vi "BlockPossibleShot.vi"(8 "error in (no error)":errorcluster, 9 "Game ref":refnum<class "Game.lvclass">, 10 "Robot in":refnum<class "Robot.lvclass">, 11 "DefendGoalTactic in":refnum<class "DefendGoalTactic.lvclass">) -> (0 "error out":errorcluster, 2 "Robot out":refnum<class "Robot.lvclass">, 3 "DefendGoalTactic out":refnum<class "DefendGoalTactic.lvclass">)   [LabVIEW 2023, in "DefendGoalTactic.lvclass"]
uses:
  DefendGoalTactic.lvclass
  Game_class/Game.lvclass
  Robot_class/Robot.lvclass
  Game_class/Game.lvclass/Game.ctl
  Object_class/Object.lvclass/Object.ctl
  Field_class/Field.lvclass/Field.ctl
  Robot_class/Robot.lvclass/Robot.ctl
  Game_class/Read BallRef.vi
  Game_class/Read FieldRef.vi
  Field_class/Read ourGoalPosition.vi
  Object_class/Read position(x,y).vi
  Robot_class/Write dest_orientation.vi
  Robot_class/Write dest_x.vi
  Robot_class/Write dest_y.vi
  Ball_class/Ball.lvclass
  C:/Users/ebert/Desktop/roboime/SSL_AI/Object_class/Object.lvclass
  Field_class/Field.lvclass
  <vilib>/Analysis/NI_AALPro.lvlib
  Utilities_class/Utilities.lvclass
  <vilib>/Analysis/coordinate.llb/2D Cartesian Coordinate Rotation (Scalar).vi
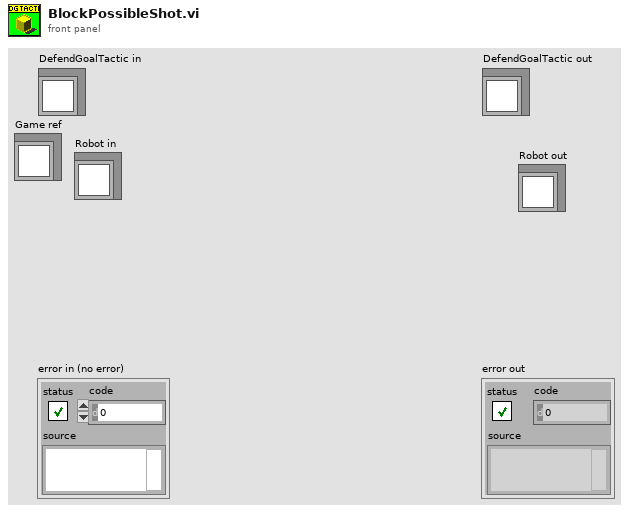
[diagram p1: front panel]
types:
  T1 = typedef "NewParameters.ctl" = cluster{"PenaltyDistance":dbl, "DistanceAttackerToBackBall":dbl, "Division":enum16{"Div B", "Div A"}, "DistanceToAvoidyEnemyRobot":dbl, "BallPlacementDistance":dbl, "DisatanceBehindBallToStealBall":dbl, "MaxDistanceToPositionKickoff":dbl, "BlockEnemyTarget":bool, "MaxStopVAng":dbl, "DistanceMarkerToEnemy":dbl, "IgnoreDribblerContact":bool, "DistanceToBeginEnemyPosession":dbl, "GoToBallWhenEnemyNotMoving":bool, "EnemyDistanceToReduceVelocity":dbl, "TurnOnEnemyDistanceToReduceVelocity":bool, "EnemyDistanceToShootOutBall":dbl, "DefenseKickBall":bool, "MoreKickToGoal? (0-0.3)":dbl, "ChipKickInEnemyField":bool, "ShootOutRobotId":dbl, "FieldLenghtDenominatorInShootOut":dbl, "AdjustPositionInBallPlacement":bool, "PowerGodPass":dbl, "VelocityAbortEnemyPos":dbl, "MaxDistToBeginPass":dbl, "MinDistToBeginPass":dbl, "VelocityInDirects":dbl, "BadDribblerIDs":i32[], "NewKickToDistanceAroundBall":dbl, "PowerAvoidColisionMarker":dbl, "DistanceToAvoidColisionMarker":dbl, "AvoidBallKick":dbl, "DistanceTryKick":dbl, "SuicideKickDIstance":dbl, "AdjustFirstKickDistance":dbl, "AvoidAimLessKick":dbl, "DistanceToAvoidyEnemyShootRobot ":dbl, "NumberOfMarkers":dbl, "PotField":bool, "PIDLateral":bool, "MinDistanceFirstKickX":dbl, "MinDistanceFirstKickY":dbl, "FractionOfDistToTouchGround\nAfterChipKick":dbl, "FractionOfKickxWhen\nComposedWithKickz":dbl, "Style":T2, "MoveInTurnState":bool, "DistFromEnemyToConsider\nMoveInTurnState":dbl, "CascadePID":bool, "TurnAroundParameters":cluster{"Radius":dbl, "Multiplier":dbl, "ChordAngle":dbl}, "SafeDriveVel":dbl, "DistanceToGoToBackBall":dbl, "minDistanceToNotFinish\nEnemyPossession":dbl, "OneTouchShot":cluster{"angleFactor":dbl, "maxAngle":dbl, "Attack":bool, "Defense":bool}, "OpenAngleToGoal":cluster{"minAngle":dbl, "maxAngle":dbl, "minEvaluation":dbl}, "ShotInterception":cluster{"shotSpeed":dbl, "minEnemySpeed":dbl, "maxEnemySpeed":dbl, "minEvaluation":dbl}, "AllyTeamArray":T3[], "maxDefendersNumber":i32, "Zone":cluster{"GuardPositionArray":dbl[][], "ZoneMidField":dbl[], "CenterForwardWidth":dbl}, "MinEvaluationToShoot":dbl, "PassInterception":cluster{"maxPassSpeed":dbl, "minPassSpeed":dbl, "minEnemySpeed":dbl, "chipPassDistance":dbl, "chipPassEvaluation":dbl, "minEvaluation":dbl, "maxEnemySpeed":dbl}, "PassDistance":cluster{"maxDistance":dbl, "minDistance":dbl}, "receiverSpeed":dbl, "maxBallSpeed":dbl, "slackTime":dbl, "Turning radius":dbl, "Turning v_ang":dbl, "AlignError":cluster{"Distance":dbl, "Orientation":dbl, "V_norm(m/s)":dbl, "V_ang (rad/s)":dbl}, "RobotRadius":dbl, "KickerDistance":dbl, "keeper angle  to cover goalpost":dbl}
  T2 = typedef "Style.ctl" = enum16{"Insanity", "Offensive", "Defensive"}
  T3 = typedef "AllyTeam.ctl" = enum16{"Keeper", "Defender", "Attacker"}
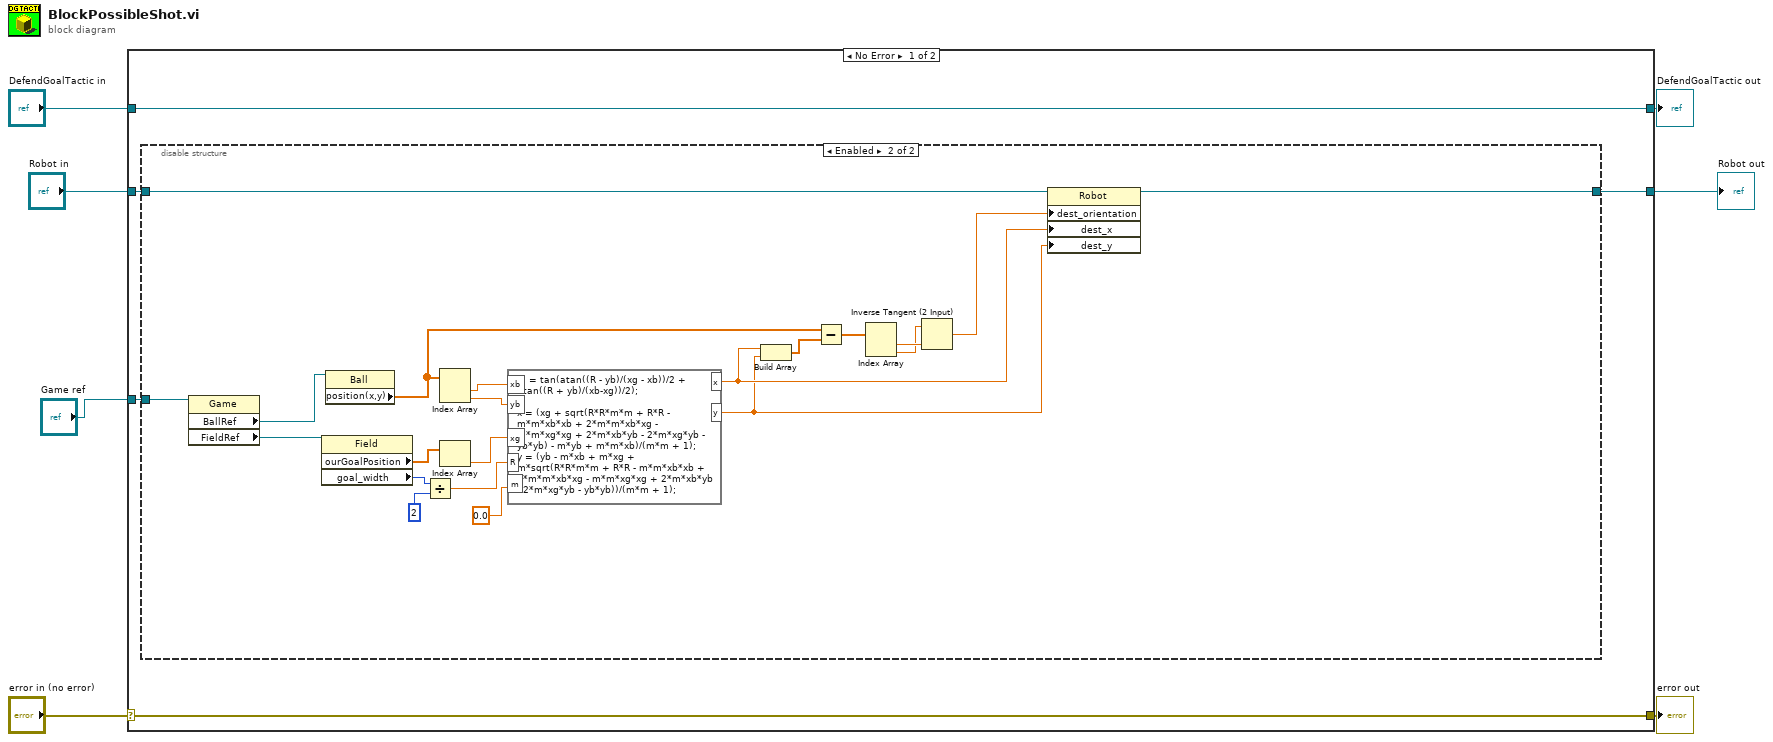
[diagram p0: block diagram]
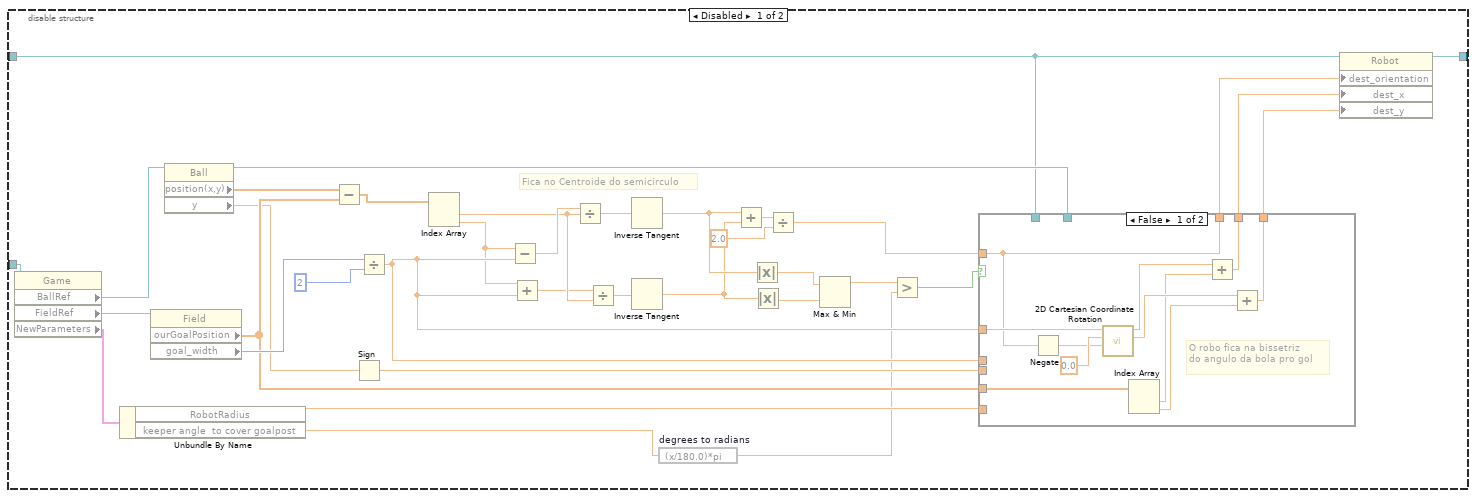
[diagram p2: hidden frame]
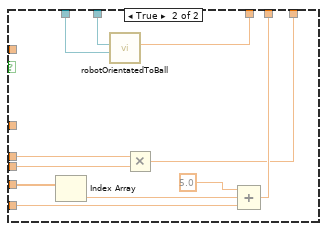
[diagram p3: hidden frame]
diagram:
  n1 = case shown="No Error" "error in (no error)" {
    selector: "error in (no error)" -> [w11 w94]
    tunnel: [w11 w94] -> w6
    tunnel: [w12 w93] -> w4
    tunnel: "DefendGoalTactic in" -> [w12 w93]
    tunnel: "Game ref" -> [w10 _]
    tunnel: "Robot in" -> [w8 w92]
    tunnel: [w9 w92] -> w1
    frame No Error {
      n2 = disable-structure shown="Enabled" {
        disable-tunnel: w10 -> [w23 w91]
        disable-tunnel: [w22 w75] -> w9
        disable-tunnel: w8 -> [w21 w76]
        frame Disabled {
          # "Fica no Centroide do semicirculo"
          n3 = property class="Game"(reference=w23) -> ("BallRef"=w48:refnum<class "Ball.lvclass">, "FieldRef"=w47:refnum<class "Field.lvclass">, "NewParameters"=w29:T1)  [unwired: 1 in, 2 out]
          n4 = Unbundle By Name(w29) -> ("RobotRadius"=w28:dbl, "keeper angle  to cover goalpost"=w13:dbl)
          n5 = property class="Field"(reference=w47) -> ("ourGoalPosition"=w35:dbl[], "goal_width"=w36:i32)  [unwired: 1 in, 2 out]
          n6 = property class="Ball"(reference=w48) -> (reference out=w30:refnum<class "Ball.lvclass">, "position(x,y)"=w46:dbl[], "y"=w25:dbl)  [unwired: 1 in, 1 out]
          n7 = Subtract(x=w46, y=w35) -> (x-y=w44:dbl[])
          n8 = Sign(1:w25) -> (0:w24:dbl)
          n9 = Divide(x=w36, y=2) -> (x/y=w27:dbl)
          n10 = Index Array(array=w44) -> (element #1=w42:dbl, element #2=w26:dbl)  [unwired: 2 in]
          n11 = Subtract(x=w26, y=w27) -> (x-y=w43:dbl)
          n12 = Add(x=w26, y=w27) -> (x+y=w41:dbl)
          n13 = Divide(x=w43, y=w42) -> (x/y=w45:dbl)
          n14 = Divide(x=w41, y=w42) -> (x/y=w40:dbl)
          n15 = Inverse Tangent(1:w45) -> (0:w20:dbl)
          n16 = Inverse Tangent(1:w40) -> (0:w19:dbl)
          n17 = expression code="(x/180.0)*pi" "degrees to radians"(w13) -> (w15:dbl)
          n18 = Add(x=w20, y=w19) -> (x+y=w38:dbl)
          n19 = Absolute Value(x=w20) -> (abs(x)=w18:dbl)
          n20 = Absolute Value(x=w19) -> (abs(x)=w17:dbl)
          n21 = Divide(x=w38, y=2.0) -> (x/y=w32:dbl)
          n22 = Max & Min(x=w18, y=w17) -> (max(x,y)=w16:dbl)  [unwired: 1 out]
          n23 = Greater?(x=w16, y=w15) -> (0:w14:bool)
          n24 = case shown="False" w14 {
            tunnel: w27 -> [w58 _]
            tunnel: w35 -> [w57 w67]
            tunnel: [w51 w64] -> w34
            tunnel: [w50 w61] -> w33
            tunnel: w32 -> [w49 _]
            tunnel: [w49 w69] -> w31
            tunnel: w30 -> [_ w70]
            tunnel: w28 -> [_ w68]
            tunnel: w27 -> [_ w62]
            tunnel: w24 -> [_ w63]
            tunnel: w21 -> [_ w60]
            frame False {
              # "O robo fica na bissetriz \ndo angulo da bola pro gol"
              n25 = Negate(x=w49) -> (-x=w54:dbl)
              n26 = call-poly <vilib>:"2D Cartesian Coordinate Rotation.vi"("theta"=w54, "y"=0.0, "x"=w58) -> ("y out"=w55:dbl, "x out"=w56:dbl)  [unwired: 6 in, 1 out]
              n27 = Index Array(array=w57) -> (element #1=w53:dbl, element #2=w52:dbl)  [unwired: 2 in]
              n28 = Add(x=w56, y=w53) -> (x+y=w51:dbl)
              n29 = Add(x=w55, y=w52) -> (x+y=w50:dbl)
            }
            frame True {
              n30 = Index Array(array=w67) -> (element=w66:dbl)  [unwired: 1 in]
              n31 = call "robotOrientatedToBall.vi"("Robot"=w60, "BallRef"=w70) -> ("Orientation"=w69:dbl)  [unwired: 7 in, 2 out]
              n32 = Multiply(x=w62, y=w63) -> (x*y=w61:dbl)
              n33 = Compound Arithmetic op=ADD(5.0 ("value"), w66, w68) -> (w64:dbl)
            }
          }
          n34 = property class="Robot"(reference=w21, "dest_orientation"=w31, "dest_x"=w34, "dest_y"=w33) -> (reference out=w22:refnum<class "Robot.lvclass">)  [unwired: 1 in, 1 out]
        }
        frame Enabled {
          n35 = property class="Game"(reference=w91) -> ("BallRef"=w89:refnum<class "Ball.lvclass">, "FieldRef"=w90:refnum<class "Field.lvclass">)  [unwired: 1 in, 2 out]
          n36 = property class="Field"(reference=w90) -> ("ourGoalPosition"=w86:dbl[], "goal_width"=w84:i32)  [unwired: 1 in, 2 out]
          n37 = property class="Ball"(reference=w89) -> ("position(x,y)"=w80:dbl[])  [unwired: 1 in, 2 out]
          n38 = Divide(x=w84, y=2) -> (x/y=w82:dbl)
          n39 = Index Array(array=w80) -> (element #1=w88:dbl, element #2=w87:dbl)  [unwired: 2 in]
          n40 = Index Array(array=w86) -> (element=w85:dbl)  [unwired: 1 in]
          n41 = formula code="m = tan(atan((R - yb)/(xg - xb))/2 + atan((R + yb)/(xb-xg))/2);\n\nx = (xg + sqrt(R*R*m*m + R*R - m*m*xb*xb + 2*m*m*xb*xg - m*m*xg*xg + 2*m*xb*yb - 2*m*xg*yb - yb*yb) - m*yb + m*m*xb)/(m*m + 1);\ny = (yb - m*xb + m*xg + m*sqrt(R*R*m*m + R*R - m*m*xb*xb + 2*m*m*xb*xg - m*m*xg*xg + 2*m*xb*yb - 2*m*xg*yb - yb*yb))/(m*m + 1);"("xb"=w88, "yb"=w87, "xg"=w85, "R"=w82, "m"=0.0 ("input variable")) -> ("x"=w73:dbl, "y"=w72:dbl)
          n42 = Build Array(w73, w72) -> (w81:dbl[])
          n43 = Subtract(x=w80, y=w81) -> (x-y=w79:dbl[])
          n44 = Index Array(array=w79) -> (element #1=w78:dbl, element #2=w77:dbl)  [unwired: 2 in]
          n45 = Inverse Tangent (2 Input)(1:w78, 2:w77) -> (0:w74:dbl)
          n46 = property class="Robot"(reference=w76, "dest_orientation"=w74, "dest_x"=w73, "dest_y"=w72) -> (reference out=w75:refnum<class "Robot.lvclass">)  [unwired: 1 in, 1 out]
        }
      }
    }
    frame Error {
    }
  }
  "error out" <- w6
  "DefendGoalTactic out" <- w4
  "Robot out" <- w1
